vi "ScanPoints (host).vi"(10 "Points":i32[][](array[numeric]), 11 "FPGA VI Reference Out":T1) -> ()   [LabVIEW 2012]
uses:
  AODRef.ctl
  <vilib>/Utility/error.llb/Error Cluster From Error Code.vi
  <vilib>/rvi/errors/niLvFpgaAdjustHostInterfaceError.vi
  <vilib>/rvi/interface/nirviMethod/nirviMethod.xnode
  FPGA Bitfiles/AodScanner_FPGATarget_AODControl(FPGA)_HzWc4w5qqfg.lvbitx
  <vilib>/FPGAPlugInAG/PXIe-7965R/niLvFpga_WriteFifo_PXIe-7965R.vi
  <vilib>/rvi/errors/niLvFpgaMergeErrorWithErrorCode.vi
panel:
  out "Empty Elements Remaining":u32
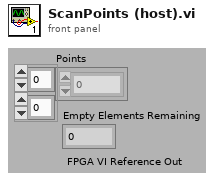
[diagram p1: front panel]
types:
  T1 = typedef "AODRef.ctl" = refnum<k20>
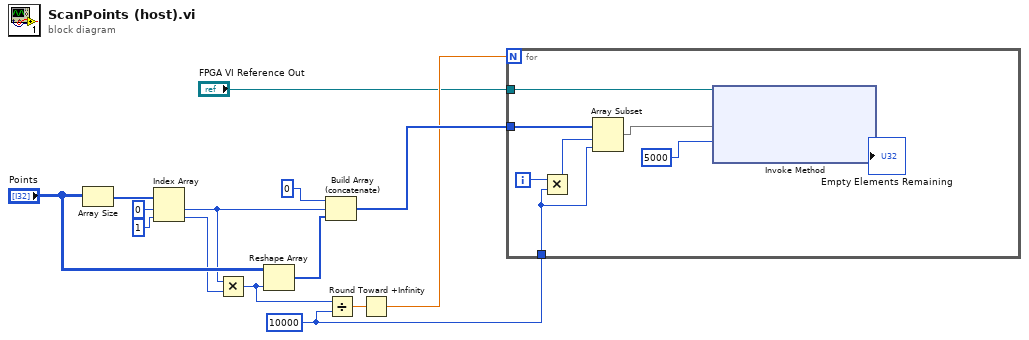
[diagram p0: block diagram]
diagram:
  w3 = 10000 ("y")
  n1 = Array Size(array="Points") -> (size(s)=w14:i32[])
  n2 = Index Array(array=w14, index #1=0 ("index"), index #2=1 ("index")) -> (element #1=w8:i32, element #2=w7:i32)
  n3 = Multiply(x=w8, y=w7) -> (x*y=w6:i32)
  n4 = Reshape Array("Points", w6) -> (w2:i32[])
  n5 = Build Array (concatenate)(0, w8, w2) -> (w9:i32[])
  n6 = Divide(x=w6, y=w3) -> (x/y=w5:dbl)
  n7 = Round Toward +Infinity(x=w5) -> (ceil(x): smallest int >= x=w4:dbl)
  n8 = for {
    N: w4 -> [_]
    tunnel: w9 -> [w18]
    tunnel: "FPGA VI Reference Out" -> [w20]
    tunnel: w3 -> [w16]
    i -> [w19]
    n9 = Multiply(x=w19, y=w16) -> (x*y=w17:i32)
    n10 = Array Subset(array=w18, index=w17, length=w16) -> (w15:i32[])
    n11 = xnode "Invoke Method"("FPGA VI Reference In"=w20, "Data"=w15, "Timeout (ms)"=5000) -> ("Empty Elements Remaining"=→"Empty Elements Remaining":u32)  [unwired: 1 in, 2 out]
  }
